vi "img test12(get XY out).vi"() -> ()   [LabVIEW 2009]
uses:
  <vilib>/vision/NI_Vision_Development_Module.lvlib
panel:
  in  "Boolean":bool
  out "Waveform Chart":cluster{"f":dbl, "f":dbl}(graph)
  out "Image 4":T1(plugin-control)
  in  "frame jump":i32=3
  in  "speed":u32(slide)=200 scale=1000.0..0.0
  in  "start":i32(slide) step=219843704 scale=0.0..124012.0
  out "Image 3":T1(plugin-control)
  out "Image 2":T1(plugin-control)
  in  "AVI Path":path=path "C:/Users/Kokum Weeratunga/Desktop/img processing/ChongWei vs LinDan (japan open 2010).avi"
  # "thilini hendahewa"
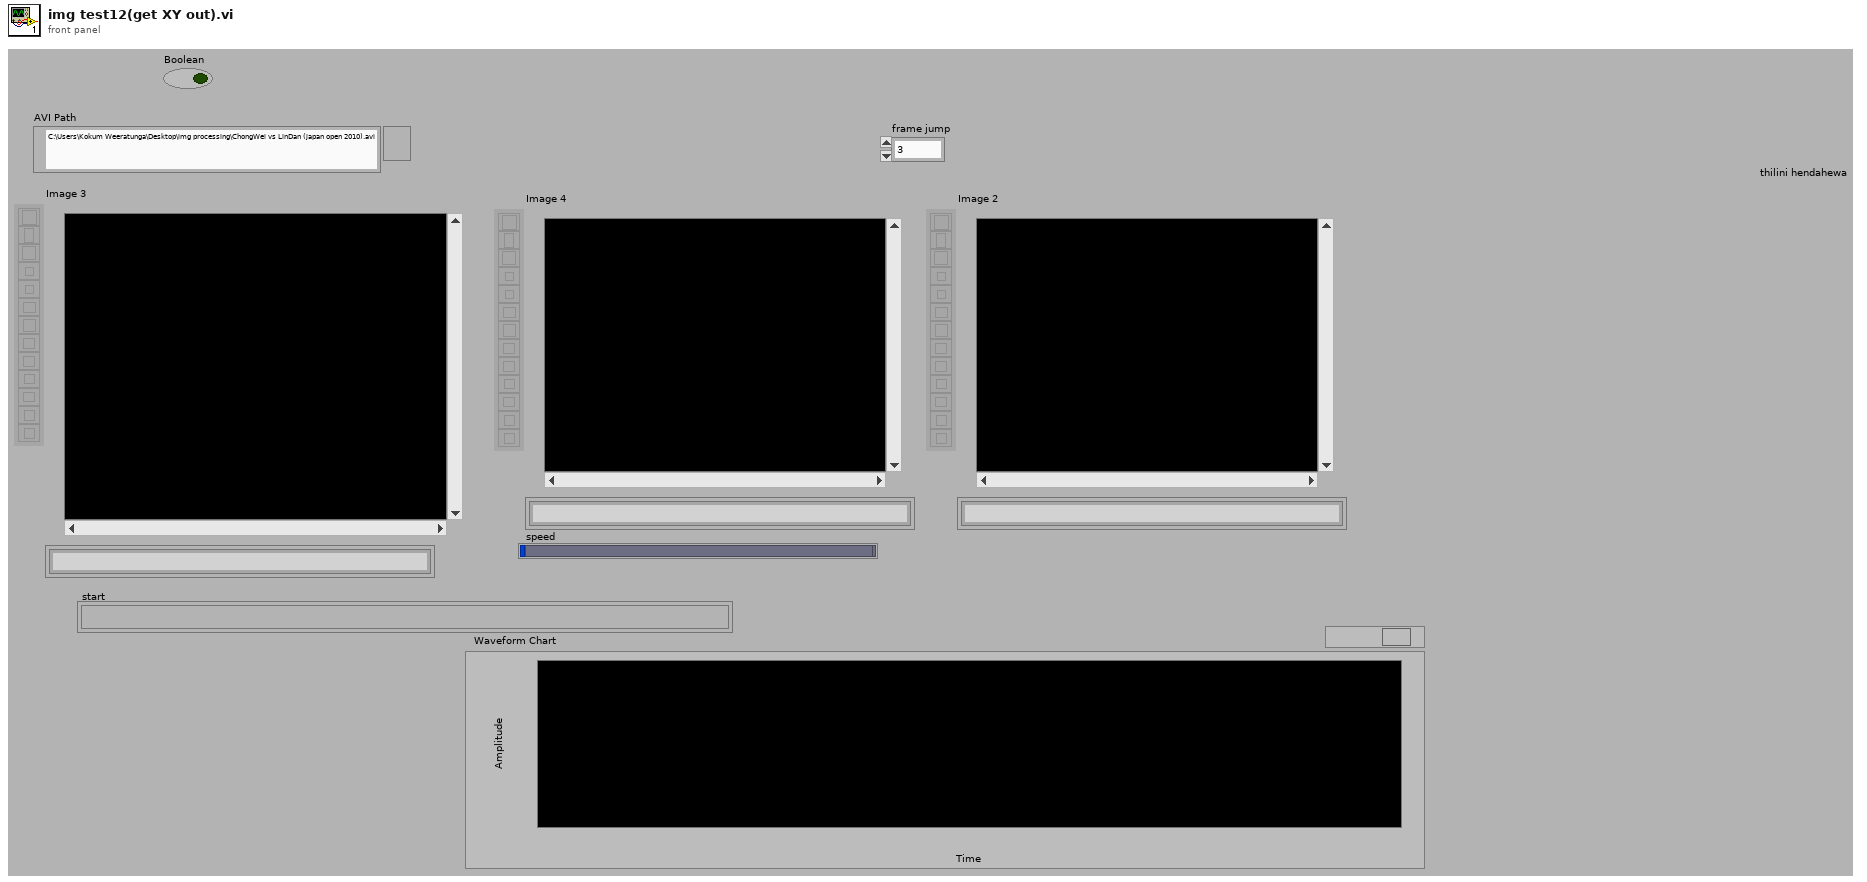
[diagram p1: front panel]
types:
  T1 = typedef "IMAQ Image.ctl" = refnum<image>
  T2 = typedef "Image Type" = u32
  T3 = typedef "AviRefnum.ctl" = refnum<k1>
  T4 = typedef "Particle Parameters" = i32
  T5 = cluster{"Numeric":dbl, "Numeric":dbl, "Numeric":dbl, "Numeric":dbl}
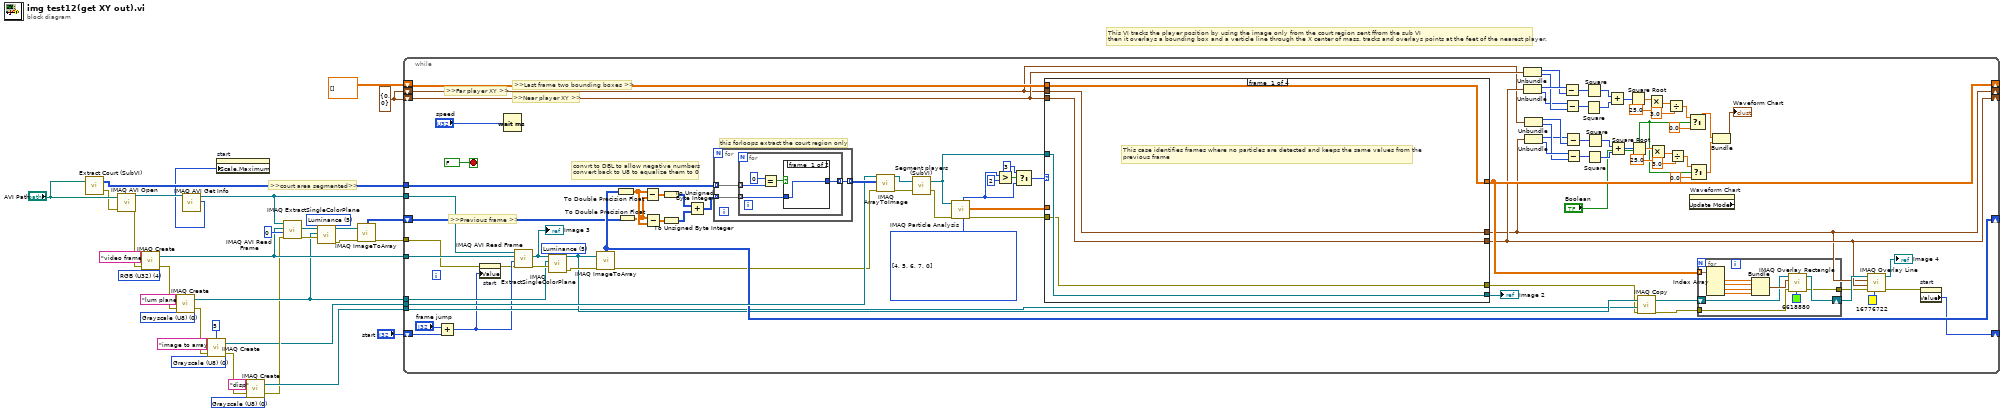
[diagram p0: block diagram]
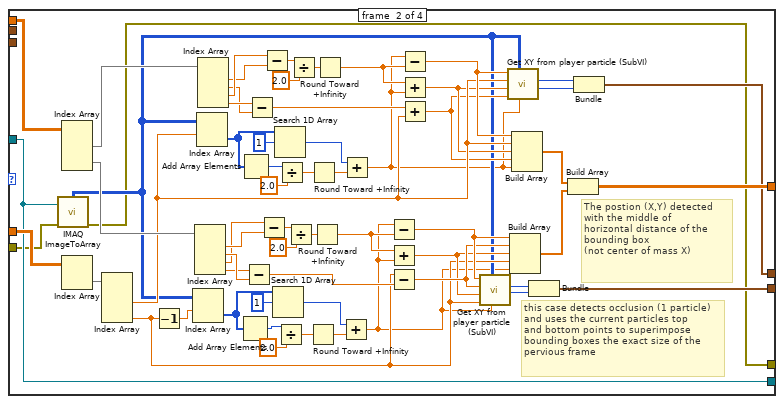
[diagram p2: hidden frame]
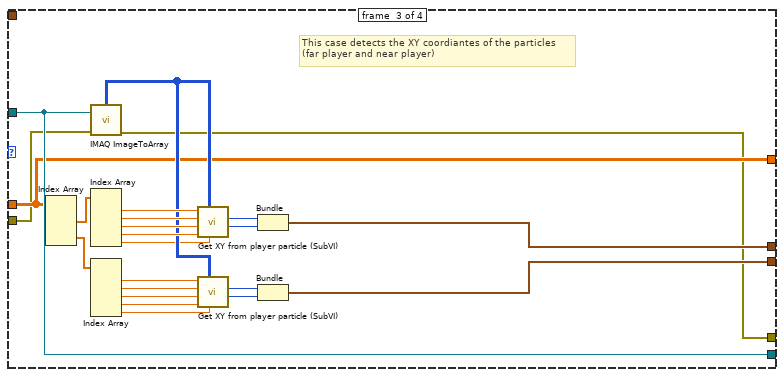
[diagram p3: hidden frame]
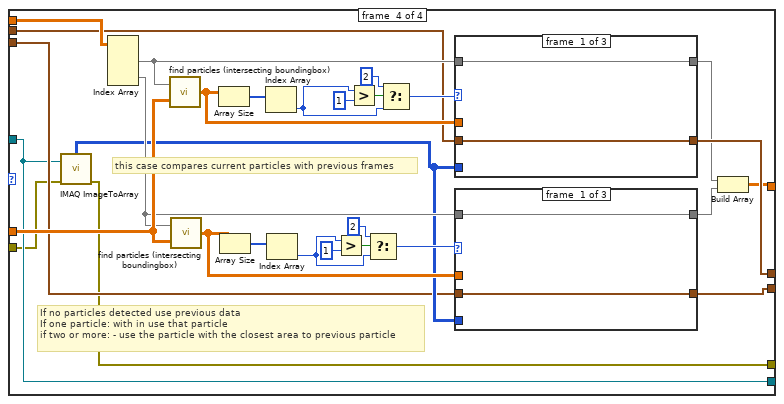
[diagram p4: hidden frame]
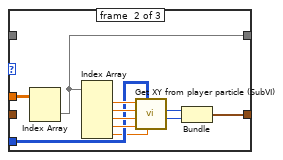
[diagram p5: hidden frame]
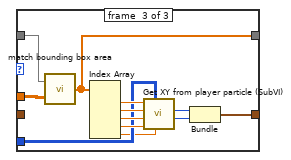
[diagram p6: hidden frame]
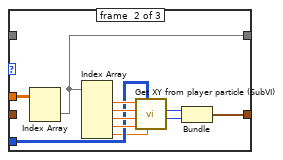
[diagram p7: hidden frame]
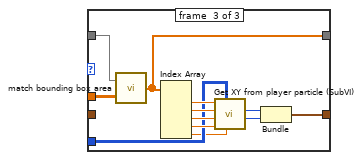
[diagram p8: hidden frame]
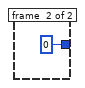
[diagram p9: hidden frame]
diagram:
  w6 = cluster{"X coordinate":i32, "Y coordinate":i32} {"X coordinate"=0, "Y coordinate"=0}
  w19 = T2 0 items=["Grayscale (U8)", "Grayscale (I16)", "Grayscale (SGL)", "Complex (CSG)", "RGB (U32)", "HSL (U32)", "RGB (U64)", "Grayscale (U16)"] ("Image Type")
  w26 = 5 items=["Red", "Green", "Blue", "Hue", "Saturation", "Luminance", "Value", "Intensity"] ("Color Plane")
  w28 = T2 0 items=["Grayscale (U8)", "Grayscale (I16)", "Grayscale (SGL)", "Complex (CSG)", "RGB (U32)", "HSL (U32)", "RGB (U64)", "Grayscale (U16)"] ("Image Type")
  w32 = T2 0 items=["Grayscale (U8)", "Grayscale (I16)", "Grayscale (SGL)", "Complex (CSG)", "RGB (U32)", "HSL (U32)", "RGB (U64)", "Grayscale (U16)"] ("Image Type")
  w30 = T2 4 items=["Grayscale (U8)", "Grayscale (I16)", "Grayscale (SGL)", "Complex (CSG)", "RGB (U32)", "HSL (U32)", "RGB (U64)", "Grayscale (U16)"] ("Image Type")
  # ">>court area segmented>>"
  # "This VI tracks the player position by using the image only from the court region sent ffrom the sub VI\nthen it overlays a bounding box and a verticle line through the X center of mass. tracks and overlays points at the feet of the nearest player."
  n1 = call "Extract Court (SubVI).vi"("AVI Path"="AVI Path") -> ("error out"=w34:errorcluster, "Court pixels out"=w9:u8[][])  [unwired: 1 in]
  n2 = call "IMAQ AVI Open"("error in (no error)"=w34, "AVI Path"="AVI Path") -> ("error out"=w15:errorcluster, "Avi Refnum"=w4:T3)  [unwired: 8 in]
  n3 = call "IMAQ Create"("Image Name"="video frame", "Image Type"=w30, "error in (no error)"=w15) -> ("New Image"=w23:T1, "error out"=w14:errorcluster)  [unwired: 2 in]
  n4 = call "IMAQ Create"("Image Name"="lum plane", "Image Type"=w32, "error in (no error)"=w14) -> ("New Image"=w22:T1, "error out"=w13:errorcluster)  [unwired: 2 in]
  n5 = call "IMAQ AVI Get Info"("Avi Refnum"=w4) -> ("Number of Frames"=w2:u32, "Avi Refnum (duplicate)"=w3:T3)  [unwired: 6 in, 3 out]
  n6 = call "IMAQ Create"("Border Size"=5, "Image Name"="image to array", "Image Type"=w28, "error in (no error)"=w13) -> ("New Image"=w8:T1, "error out"=w12:errorcluster)  [unwired: 1 in]
  n7 = property on="start" class="Slide (strict)"("Scale.Maximum"=w2) -> ()  [unwired: 2 in, 2 out]
  n8 = call "IMAQ Create"("Image Name"="disp", "Image Type"=w19, "error in (no error)"=w12) -> ("New Image"=w17:T1, "error out"=w11:errorcluster)  [unwired: 2 in]
  n9 = call "IMAQ AVI Read Frame"("error in (no error)"=w11, "Frame Number"=u32 0, "Image"=w23, "Avi Refnum"=w3) -> ("error out"=w25:errorcluster, "Image Out"=w27:T1)  [unwired: 4 in, 2 out]
  n10 = call "IMAQ ExtractSingleColorPlane"("Color Plane"=w26, "error in (no error)"=w25, "Image Dst"=w22, "Image Src"=w27) -> ("error out"=w16:errorcluster, "Image Dst Out"=w20:T1)  [unwired: 6 in]
  n11 = call "IMAQ ImageToArray"("error in (no error)"=w16, "Image"=w20) -> ("error out"=w1:errorcluster, "Image Pixels (U8)"=w21:u8[][])  [unwired: 2 in, 3 out]
  n12 = while {
    tunnel: w3 -> [w79]
    tunnel: w23 -> [w107]
    tunnel: w9 -> [w124]
    tunnel: w22 -> [w108]
    tunnel: w8 -> [w121]
    shift-right: [w120] -> _
    shift-left: w21 -> [w119]
    tunnel: w17 -> [w86]
    shift-right: [w93] -> _
    shift-left: dbl[][] [] ("Particle Measurements (Pixels)") -> [w94]
    shift-right: [w40] -> _
    shift-left: w6 -> [w41]
    shift-right: [w60] -> _
    shift-left: w6 -> [w59]
    shift-right: [w74] -> _
    shift-left: "start" -> [w81]
    tunnel: w1 -> [w77]
    stop <- FALSE stop-if-true
    w109 = T4[] [4, 5, 6, 7, 0] items=["Center of Mass X", "Center of Mass Y", "First Pixel X", "First Pixel Y", "Bounding Rect Left", "Bounding Rect Top", "Bounding Rect Right", "Bounding Rect Bottom", "Max Feret Diameter Start X", "Max Feret Diameter Start Y", "Max Feret Diameter End X", "Max Feret Diameter End Y", "Max Horiz. Segment Length Left", "Max Horiz. Segment Length Right", "Max Horiz. Segment Length Row", "-", "Bounding Rect Width", "Bounding Rect Height", "Bounding Rect Diagonal", "Perimeter", "Convex Hull Perimeter", "Holes' Perimeter", "Max Feret Diameter", "Equivalent Ellipse Major Axis", "Equivalent Ellipse Minor Axis", "Equivalent Ellipse Minor Axis (Feret)", "Equivalent Rect Long Side", "Equivalent Rect Short Side", "Equivalent Rect Diagonal", "Equivalent Rect Short Side (Feret)", "Average Horiz. Segment Length", "Average Vert. Segment Length", "Hydraulic Radius", "Waddel Disk Diameter", "-", "Area", "Holes' Area", "Particle & Holes' Area", "Convex Hull Area", "Image Area", "-", "Number of Holes", "Number of Horiz. Segments", "Number of Vert. Segments", "-", "Orientation", "Max Feret Diameter Orientation", "-", "% Area/Image Area", "% Area/(Particle & Holes' Area)", "Ratio of Equivalent Ellipse Axes", "Ratio of Equivalent Rect Sides", "-", "Elongation Factor", "Compactness Factor", "Heywood Circularity Factor", "Type Factor", "-", "Sum X", "Sum Y", "Sum XX", "Sum XY", "Sum YY", "Sum XXX", "Sum XXY", "Sum XYY", "Sum YYY", "-", "Moment of Inertia XX", "Moment of Inertia XY", "Moment of Inertia YY", "Moment of Inertia XXX", "Moment of Inertia XXY", "Moment of Inertia XYY", "Moment of Inertia YYY", "Norm. Moment of Inertia XX", "Norm. Moment of Inertia XY", "Norm. Moment of Inertia YY", "Norm. Moment of Inertia XXX", "Norm. Moment of Inertia XXY", "Norm. Moment of Inertia XYY", "Norm. Moment of Inertia YYY", "Hu Moment 1", "Hu Moment 2", "Hu Moment 3", "Hu Moment 4", "Hu Moment 5", "Hu Moment 6", "Hu Moment 7"] ("Pixel Measurements")
    w125 = 5 items=["Red", "Green", "Blue", "Hue", "Saturation", "Luminance", "Value", "Intensity"] ("Color Plane")
    # ">>Last frame two bounding boxes >>"
    # ">>Far player XY >>"
    # ">>Near player XY >>"
    # ">>Previous frame >>"
    # "convrt to DBL to allow negative numbers\nconvert back to U8 to equalize them to 0"
    # "this forloops extract the court region only"
    n13 = Add(x="frame jump", y=w81) -> (x+y=w78:i32)
    n14 = property on="start" class="Slide (strict)"(error in=w77, "Value"=w78) -> (error out=w76:errorcluster)  [unwired: 1 in, 1 out]
    n15 = Wait (ms)(milliseconds to wait="speed") -> ()  [unwired: 1 out]
    n16 = call "IMAQ AVI Read Frame"("error in (no error)"=w76, "Frame Number"=w78, "Image"=w107, "Avi Refnum"=w79) -> ("error out"=w126:errorcluster, "Image Out"=w104:T1)  [unwired: 4 in, 2 out]
    "Image 3" <- w104
    n17 = call "IMAQ ExtractSingleColorPlane"("Color Plane"=w125, "error in (no error)"=w126, "Image Dst"=w108, "Image Src"=w104) -> ("error out"=w111:errorcluster, "Image Dst Out"=w87:T1)  [unwired: 6 in]
    n18 = call "IMAQ ImageToArray"("error in (no error)"=w111, "Image"=w87) -> ("error out"=w110:errorcluster, "Image Pixels (U8)"=w120:u8[][])  [unwired: 2 in, 3 out]
    n19 = To Double Precision Float(number=w120) -> (double precision float=w115:dbl[][])
    n20 = To Double Precision Float(number=w119) -> (double precision float=w114:dbl[][])
    n21 = Subtract(x=w115, y=w114) -> (x-y=w113:dbl[][])
    n22 = Subtract(x=w114, y=w115) -> (x-y=w112:dbl[][])
    n23 = To Unsigned Byte Integer(number=w113) -> (unsigned 8bit integer=w118:u8[][])
    n24 = To Unsigned Byte Integer(number=w112) -> (unsigned 8bit integer=w117:u8[][])
    n25 = Add(x=w118, y=w117) -> (x+y=w116:u8[][])
    n26 = for {
      tunnel: w124 -> [w308] mode=indexing
      tunnel: [w307] -> w122 mode=indexing
      tunnel: w116 -> [w306] mode=indexing
      n27 = for {
        tunnel: w308 -> [w313] mode=indexing
        tunnel: [w310] -> w307 mode=indexing
        tunnel: w306 -> [w309] mode=indexing
        n28 = Equal?(x=u8 0, y=w313) -> (x = y?=w311:bool)
        n29 = case shown="True" w311 {
          tunnel: [w314 u8 0 ("x")] -> w310
          tunnel: w309 -> [w314 _]
          frame #0 {
          }
          frame #1 {
          }
        }
      }
    }
    n30 = call "IMAQ ArrayToImage"("error in (no error)"=w110, "Image Pixels (U8)"=w122, "Image"=w121) -> ("error out"=w105:errorcluster, "Image Out"=w106:T1)  [unwired: 7 in]
    n31 = call "Segment players (SubVI).vi"("error In"=w105, "Image In"=w106) -> ("error out"=w98:errorcluster, "Image Out"=w96:T1)
    n32 = call "IMAQ Particle Analysis"("error in (no error)"=w98, "Pixel Measurements"=w109, "Image"=w96) -> ("error out"=w97:errorcluster, "Particle Measurements (Pixels)"=w95:dbl[][], "Number of Particles"=w100:i32)  [unwired: 3 in, 3 out]
    n33 = Greater?(x=w100, y=2) -> (0:w103:bool)
    n34 = Select(t=3 ("y"), s=w103, f=w100) -> (s? t:f=w99:i32)
    n35 = case shown="1" w99 {
      tunnel: [w141 w168 w222 w232] -> w91
      tunnel: w95 -> [_ w203 w208 w252]
      tunnel: w97 -> [w138 w144 w205 w228]
      tunnel: w96 -> [w141 w168 w222 w232]
      tunnel: [w139 w152 w210 w234] -> w60
      tunnel: [w140 w159 w209 w233] -> w40
      tunnel: [w142 w169 w208 w229] -> w93
      tunnel: w94 -> [w142 w193 _ w255]
      tunnel: w41 -> [w140 _ _ w240]
      tunnel: w59 -> [w139 _ _ w235]
      tunnel: [w138 w143 w204 w227] -> w84
      frame #0 {
        # "This case identifies frames where no particles are detected and keeps the same values from the\nprevious frame"
      }
      frame #1 {
        # "The postion (X,Y) detected with the middle of \nhorizontal distance of the bounding box\n(not center of mass X)"
        # "this case detects occlusion (1 particle)\nand uses the current particles top \nand bottom points to superimpose \nbounding boxes the exact size of the \npervious frame"
        n36 = call "IMAQ ImageToArray"("error in (no error)"=w144, "Image"=w168) -> ("error out"=w143:errorcluster, "Image Pixels (U8)"=w151:u8[][])  [unwired: 2 in, 3 out]
        n37 = Index Array(array=w193) -> (element #1=w201:dbl[], element #2=w173:dbl[])  [unwired: 4 in]
        n38 = Index Array(array=w203) -> (element=w202:dbl[])  [unwired: 2 in]
        n39 = Index Array(array=w202) -> (element #2=w164:dbl, element #4=w155:dbl)  [unwired: 4 in, 2 out]
        n40 = Decrement(x=w155) -> (x-1=w166:dbl)
        n41 = Index Array(array=w151, index (row)=w166) -> (element=w188:u8[])  [unwired: 1 in]
        n42 = Index Array(array=w173) -> (element #1=w177:dbl, element #2=w180:dbl, element #3=w176:dbl, element #4=w179:dbl)  [unwired: 4 in]
        n43 = Index Array(array=w151, index (row)=w164) -> (element=w181:u8[])  [unwired: 1 in]
        n44 = Index Array(array=w201) -> (element #1=w197:dbl, element #2=w194:dbl, element #3=w198:dbl, element #4=w195:dbl)  [unwired: 4 in]
        n45 = Add Array Elements(numeric array=w188) -> (sum=w189:u8)
        n46 = Add Array Elements(numeric array=w181) -> (sum=w185:u8)
        n47 = Subtract(x=w179, y=w180) -> (x-y=w167:dbl)
        n48 = Subtract(x=w195, y=w194) -> (x-y=w172:dbl)
        n49 = Subtract(x=w176, y=w177) -> (x-y=w175:dbl)
        n50 = Subtract(x=w198, y=w197) -> (x-y=w199:dbl)
        n51 = Search 1D Array(1D array=w188, element=u8 1) -> (index of element=w187:i32)  [unwired: 1 in]
        n52 = Search 1D Array(1D array=w181, element=u8 1) -> (index of element=w186:i32)  [unwired: 1 in]
        n53 = Divide(x=w189, y=2.0) -> (x/y=w190:dbl)
        n54 = Divide(x=w185, y=2.0) -> (x/y=w184:dbl)
        n55 = Divide(x=w175, y=2.0) -> (x/y=w178:dbl)
        n56 = Divide(x=w199, y=2.0) -> (x/y=w196:dbl)
        n57 = Round Toward +Infinity(x=w190) -> (ceil(x): smallest int >= x=w149:dbl)
        n58 = Round Toward +Infinity(x=w184) -> (ceil(x): smallest int >= x=w148:dbl)
        n59 = Round Toward +Infinity(x=w178) -> (ceil(x): smallest int >= x=w150:dbl)
        n60 = Round Toward +Infinity(x=w196) -> (ceil(x): smallest int >= x=w147:dbl)
        n61 = Add(x=w187, y=w149) -> (x+y=w145:dbl)
        n62 = Add(x=w186, y=w148) -> (x+y=w146:dbl)
        n63 = Subtract(x=w145, y=w150) -> (x-y=w158:dbl)
        n64 = Add(x=w150, y=w145) -> (x+y=w156:dbl)
        n65 = Subtract(x=w155, y=w167) -> (x-y=w157:dbl)
        n66 = Subtract(x=w146, y=w147) -> (x-y=w165:dbl)
        n67 = Add(x=w147, y=w146) -> (x+y=w163:dbl)
        n68 = Add(x=w172, y=w164) -> (x+y=w162:dbl)
        n69 = call "Get XY from player particle (SubVI).vi"("Center of mass X"=w145, "Image in Pixels (U8)"=w151, "Particle bounding rect bottom"=w155, "Particle bounding rect right"=w156, "Particle bounding rect top"=w157, "Particle bounding rect left"=w158) -> ("Y coordinate"=w153:i32, "X coordinate"=w154:i32)  [unwired: 2 in]
        n70 = call "Get XY from player particle (SubVI).vi"("Center of mass X"=w146, "Image in Pixels (U8)"=w151, "Particle bounding rect bottom"=w162, "Particle bounding rect right"=w163, "Particle bounding rect top"=w164, "Particle bounding rect left"=w165) -> ("Y coordinate"=w160:i32, "X coordinate"=w161:i32)  [unwired: 2 in]
        n71 = Build Array(w158, w157, w156, w155, w145) -> (w170:dbl[])
        n72 = Build Array(w165, w164, w163, w162, w146) -> (w171:dbl[])
        n73 = Bundle("X coordinate"=w154, "Y coordinate"=w153) -> (w152:cluster{"X coordinate":i32, "Y coordinate":i32})  [unwired: 1 in]
        n74 = Build Array(w171, w170) -> (w169:dbl[][])
        n75 = Bundle("X coordinate"=w161, "Y coordinate"=w160) -> (w159:cluster{"X coordinate":i32, "Y coordinate":i32})  [unwired: 1 in]
      }
      frame #2 {
        # "This case detects the XY coordiantes of the particles\n(far player and near player)"
        n76 = Index Array(array=w208) -> (element #1=w216:dbl[], element #2=w215:dbl[])  [unwired: 4 in]
        n77 = call "IMAQ ImageToArray"("error in (no error)"=w205, "Image"=w222) -> ("error out"=w204:errorcluster, "Image Pixels (U8)"=w217:u8[][])  [unwired: 2 in, 3 out]
        n78 = Index Array(array=w216) -> (element #1=w226:dbl, element #2=w225:dbl, element #3=w224:dbl, element #4=w223:dbl, element #5=w207:dbl)  [unwired: 5 in]
        n79 = Index Array(array=w215) -> (element #1=w218:dbl, element #2=w219:dbl, element #3=w220:dbl, element #4=w221:dbl, element #5=w206:dbl)  [unwired: 5 in]
        n80 = call "Get XY from player particle (SubVI).vi"("Center of mass X"=w207, "Image in Pixels (U8)"=w217, "Particle bounding rect bottom"=w223, "Particle bounding rect right"=w224, "Particle bounding rect top"=w225, "Particle bounding rect left"=w226) -> ("Y coordinate"=w213:i32, "X coordinate"=w214:i32)  [unwired: 2 in]
        n81 = call "Get XY from player particle (SubVI).vi"("Center of mass X"=w206, "Image in Pixels (U8)"=w217, "Particle bounding rect bottom"=w221, "Particle bounding rect right"=w220, "Particle bounding rect top"=w219, "Particle bounding rect left"=w218) -> ("Y coordinate"=w211:i32, "X coordinate"=w212:i32)  [unwired: 2 in]
        n82 = Bundle("X coordinate"=w214, "Y coordinate"=w213) -> (w209:cluster{"X coordinate":i32, "Y coordinate":i32})  [unwired: 1 in]
        n83 = Bundle("X coordinate"=w212, "Y coordinate"=w211) -> (w210:cluster{"X coordinate":i32, "Y coordinate":i32})  [unwired: 1 in]
      }
      frame #3 {
        # "If no particles detected use previous data\nIf one particle: with in use that particle\nif two or more: - use the particle with the closest area to previous particle"
        # "this case compares current particles with previous frames"
        n84 = call "IMAQ ImageToArray"("error in (no error)"=w228, "Image"=w232) -> ("error out"=w227:errorcluster, "Image Pixels (U8)"=w236:u8[][])  [unwired: 2 in, 3 out]
        n85 = Index Array(array=w255) -> (element #1=w251:dbl[], element #2=w239:dbl[])  [unwired: 4 in]
        n86 = call "find particles (intersecting boundingbox).vi"("Particle Measurements in (bounding boxes)"=w252, "bounding box in"=w251) -> ("Particles within bounding box"=w250:dbl[][])
        n87 = call "find particles (intersecting boundingbox).vi"("Particle Measurements in (bounding boxes)"=w252, "bounding box in"=w239) -> ("Particles within bounding box"=w237:dbl[][])
        n88 = Array Size(array=w250) -> (size(s)=w254:i32[])
        n89 = Array Size(array=w237) -> (size(s)=w253:i32[])
        n90 = Index Array(array=w254) -> (element=w242:i32)  [unwired: 1 in]
        n91 = Index Array(array=w253) -> (element=w243:i32)  [unwired: 1 in]
        n92 = Greater?(x=w243, y=1) -> (0:w246:bool)
        n93 = Greater?(x=w242, y=1) -> (0:w247:bool)
        n94 = Select(t=2 ("y"), s=w246, f=w243) -> (s? t:f=w238:i32)
        n95 = Select(t=2 ("y"), s=w247, f=w242) -> (s? t:f=w241:i32)
        n96 = case shown="0, Default" w241 {
          tunnel: w251 -> [w282 _ w297]
          tunnel: w250 -> [_ w293 w296]
          tunnel: [w282 w284 w295] -> w231
          tunnel: w236 -> [_ w286 w299]
          tunnel: [w281 w285 w298] -> w233
          tunnel: w240 -> [w281 _ _]
          frame #0 {
          }
          frame #1 {
            n97 = Index Array(array=w293) -> (element=w284:dbl[])  [unwired: 2 in]
            n98 = Index Array(array=w284) -> (element #1=w290:dbl, element #2=w289:dbl, element #3=w288:dbl, element #4=w287:dbl, element #5=w283:dbl)  [unwired: 5 in]
            n99 = call "Get XY from player particle (SubVI).vi"("Center of mass X"=w283, "Image in Pixels (U8)"=w286, "Particle bounding rect bottom"=w287, "Particle bounding rect right"=w288, "Particle bounding rect top"=w289, "Particle bounding rect left"=w290) -> ("Y coordinate"=w291:i32, "X coordinate"=w292:i32)  [unwired: 2 in]
            n100 = Bundle("X coordinate"=w292, "Y coordinate"=w291) -> (w285:cluster{"X coordinate":i32, "Y coordinate":i32})  [unwired: 1 in]
          }
          frame #2 {
            n101 = call "match bounding box area.vi"("particle measurements (bounding box)"=w296, "bounding box in"=w297) -> ("matching bounding box"=w295:dbl[])
            n102 = Index Array(array=w295) -> (element #1=w303:dbl, element #2=w302:dbl, element #3=w301:dbl, element #4=w300:dbl, element #5=w294:dbl)  [unwired: 5 in]
            n103 = call "Get XY from player particle (SubVI).vi"("Center of mass X"=w294, "Image in Pixels (U8)"=w299, "Particle bounding rect bottom"=w300, "Particle bounding rect right"=w301, "Particle bounding rect top"=w302, "Particle bounding rect left"=w303) -> ("Y coordinate"=w304:i32, "X coordinate"=w305:i32)  [unwired: 2 in]
            n104 = Bundle("X coordinate"=w305, "Y coordinate"=w304) -> (w298:cluster{"X coordinate":i32, "Y coordinate":i32})  [unwired: 1 in]
          }
        }
        n105 = case shown="0, Default" w238 {
          tunnel: w239 -> [w257 _ w272]
          tunnel: w237 -> [_ w268 w271]
          tunnel: [w257 w259 w270] -> w230
          tunnel: w236 -> [_ w261 w274]
          tunnel: [w256 w260 w273] -> w234
          tunnel: w235 -> [w256 _ _]
          frame #0 {
          }
          frame #1 {
            n106 = Index Array(array=w268) -> (element=w259:dbl[])  [unwired: 2 in]
            n107 = Index Array(array=w259) -> (element #1=w265:dbl, element #2=w264:dbl, element #3=w263:dbl, element #4=w262:dbl, element #5=w258:dbl)  [unwired: 5 in]
            n108 = call "Get XY from player particle (SubVI).vi"("Center of mass X"=w258, "Image in Pixels (U8)"=w261, "Particle bounding rect bottom"=w262, "Particle bounding rect right"=w263, "Particle bounding rect top"=w264, "Particle bounding rect left"=w265) -> ("Y coordinate"=w266:i32, "X coordinate"=w267:i32)  [unwired: 2 in]
            n109 = Bundle("X coordinate"=w267, "Y coordinate"=w266) -> (w260:cluster{"X coordinate":i32, "Y coordinate":i32})  [unwired: 1 in]
          }
          frame #2 {
            n110 = call "match bounding box area.vi"("particle measurements (bounding box)"=w271, "bounding box in"=w272) -> ("matching bounding box"=w270:dbl[])
            n111 = Index Array(array=w270) -> (element #1=w278:dbl, element #2=w277:dbl, element #3=w276:dbl, element #4=w275:dbl, element #5=w269:dbl)  [unwired: 5 in]
            n112 = call "Get XY from player particle (SubVI).vi"("Center of mass X"=w269, "Image in Pixels (U8)"=w274, "Particle bounding rect bottom"=w275, "Particle bounding rect right"=w276, "Particle bounding rect top"=w277, "Particle bounding rect left"=w278) -> ("Y coordinate"=w279:i32, "X coordinate"=w280:i32)  [unwired: 2 in]
            n113 = Bundle("X coordinate"=w280, "Y coordinate"=w279) -> (w273:cluster{"X coordinate":i32, "Y coordinate":i32})  [unwired: 1 in]
          }
        }
        n114 = Build Array(w231, w230) -> (w229:dbl[][])
      }
    }
    "Image 2" <- w91
    n115 = Unbundle(w59) -> ("X coordinate"=w72:i32, "Y coordinate"=w71:i32)
    n116 = Unbundle(w60) -> ("X coordinate"=w73:i32, "Y coordinate"=w70:i32)
    n117 = Unbundle(w41) -> ("X coordinate"=w43:i32, "Y coordinate"=w44:i32)
    n118 = Unbundle(w40) -> ("X coordinate"=w42:i32, "Y coordinate"=w45:i32)
    n119 = Subtract(x=w73, y=w72) -> (x-y=w69:i32)
    n120 = Subtract(x=w70, y=w71) -> (x-y=w68:i32)
    n121 = Subtract(x=w42, y=w43) -> (x-y=w46:i32)
    n122 = Subtract(x=w45, y=w44) -> (x-y=w47:i32)
    n123 = Square(x=w68) -> (x^2=w66:i32)
    n124 = Square(x=w69) -> (x^2=w67:i32)
    n125 = Square(x=w47) -> (x^2=w49:i32)
    n126 = Square(x=w46) -> (x^2=w48:i32)
    n127 = Add(x=w67, y=w66) -> (x+y=w65:i32)
    n128 = Add(x=w48, y=w49) -> (x+y=w50:i32)
    n129 = Square Root(x=w65) -> (sqrt(x)=w64:dbl)
    n130 = Square Root(x=w50) -> (sqrt(x)=w51:dbl)
    n131 = call "IMAQ Copy"("error in (no error)"=w84, "Image Dst"=w86, "Image Src"=w87) -> ("error out"=w83:errorcluster, "Image Dst Out"=w85:T1)  [unwired: 3 in]
    n132 = Multiply(x=w64, y=25.0) -> (x*y=w62:dbl)
    n133 = Multiply(x=w51, y=25.0) -> (x*y=w53:dbl)
    n134 = Divide(x=w62, y=3.0) -> (x/y=w58:dbl)
    n135 = Divide(x=w53, y=3.0) -> (x/y=w55:dbl)
    n136 = Select(t=w58, s="Boolean", f=0.0) -> (s? t:f=w38:dbl)
    n137 = Select(t=w55, s="Boolean", f=0.0) -> (s? t:f=w37:dbl)
    n138 = property on="Waveform Chart" class="WFChart (strict)" props=["Update Mode"]() -> ()  [unwired: 2 in, 3 out]
    n139 = for {
      shift-right: [w129] -> w89
      shift-left: w85 -> [w133]
      tunnel: w93 -> [w131] mode=indexing
      tunnel: w83 -> [w128]
      tunnel: [w127] -> w82
      n140 = Index Array(array=w131) -> (element #1=w137:dbl, element #2=w136:dbl, element #3=w135:dbl, element #4=w130:dbl)  [unwired: 4 in]
      n141 = Bundle("Numeric"=w137, "Numeric"=w136, "Numeric"=w135, "Numeric"=w130) -> (w134:T5)  [unwired: 1 in]
      n142 = call "IMAQ Overlay Rectangle"("Color"=u32 6618880, "error in (no error)"=w128, "Rectangle"=w134, "Image"=w133) -> ("error out"=w127:errorcluster, "Image Out"=w129:T1)  [unwired: 6 in]
    }
    n143 = Bundle("f"=w38, "f"=w37) -> (→"Waveform Chart":cluster{"f":dbl, "f":dbl})  [unwired: 1 in]
    n144 = call "IMAQ Overlay Line"("Color"=u32 16776722, "error in (no error)"=w82, "End Point"=w60, "Start Point"=w40, "Image"=w89) -> ("error out"=w75:errorcluster, "Image Out"=→"Image 4":T1)  [unwired: 5 in]
    n145 = property on="start" class="Slide (strict)"(error in=w75) -> ("Value"=w74:i32)  [unwired: 1 in, 2 out]
  }
